vi "Write buffer size (S).vi"(8 "error in (no error)":errorcluster, 10 "buffer size (S)":u32, 11 "LockinDAQ":refnum<class "LockinDAQ.lvclass">) -> (0 "error out":errorcluster, 3 "LockinDAQ out":refnum<class "LockinDAQ.lvclass">)   [LabVIEW 2016, in "LockinDAQ.lvclass"]
uses:
  LockinDAQ.lvclass
  LockinDAQ.lvclass/LockinDAQ.ctl
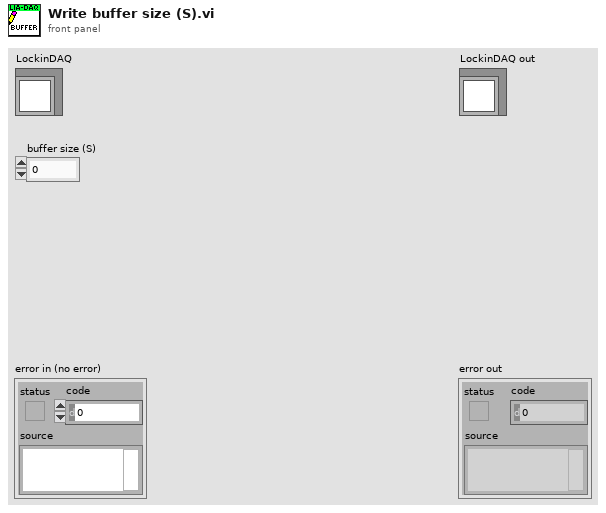
[diagram p1: front panel]
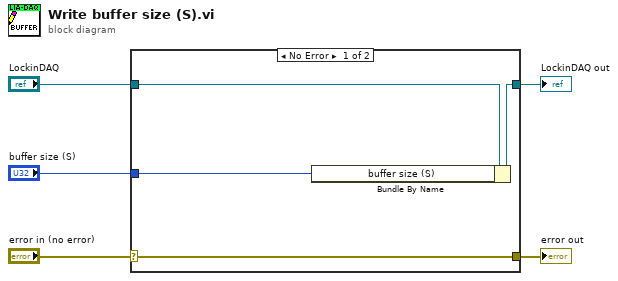
[diagram p0: block diagram]
diagram:
  n1 = case shown="No Error" "error in (no error)" {
    selector: "error in (no error)" -> [w9 w10]
    tunnel: [w9 w10] -> w4
    tunnel: [w7 w11] -> w2
    tunnel: "LockinDAQ" -> [w8 w11]
    tunnel: "buffer size (S)" -> [w6 _]
    frame No Error {
      n2 = Bundle By Name(cluster=w8, "buffer size (S)"=w6) -> (w7:refnum<class "LockinDAQ.lvclass">)
    }
    frame Error {
    }
  }
  "error out" <- w4
  "LockinDAQ out" <- w2
